vi "BKP-911x Power Supply_Create.vi"(0 "reference in":refnum<class "BKP-911x Power Supply.lvclass">, 2 "VISA resource name":refnum<visa-resource-name>, 3 "Serial Configuration":cluster{"Baud Rate":u32}={"Baud Rate"=9600} {"Baud Rate" items=["4800"=4800, "9600"=9600, "19200"=19200, "38400"=38400, "57600"=57600, "115200"=115200]}, 5 "error in (no error)":errorcluster) -> (13 "ProcessViRef":refnum<vi>, 14 "reference out":refnum<class "BKP-911x Power Supply.lvclass">, 19 "error out":errorcluster)   [LabVIEW 2018, in "BKP-911x Power Supply.lvclass"]
uses:
  BKP-911x Power Supply.lvclass
  controls/IO Signal List.ctl
  <instrlib>/BK Precision 911X Series/BK Precision 911X Series.lvlib
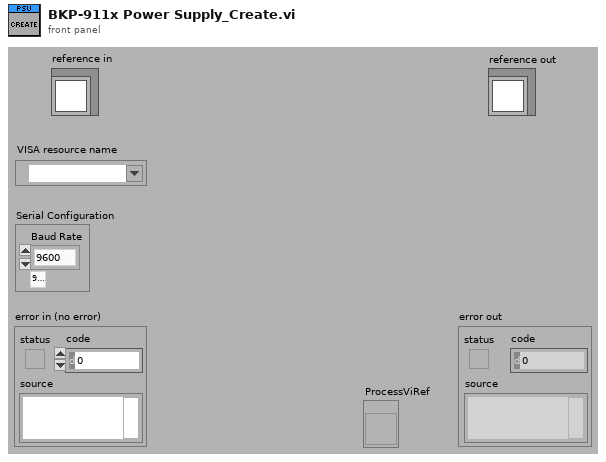
[diagram p1: front panel]
types:
  T1 = typedef "IO Signal List.ctl" = enum16{"Timestamp", "PSU_FB_U_VDC", "PSU_FB_I_AMP", "PSU_FB_W_WATT", "PSU_CMD_U_VDC", "PSU_CMD_I_AMP", "PSU_CMD_OUTPUT", "U_U_VDC", "V_U_VDC", "W_U_VDC", "U_I_AMP", "V_I_AMP", "W_I_AMP", "LCR_PRIMARY", "LCR_SECONDARY", "UV_R_mOhm", "UW_R_mOhm", "VW_R_mOhm", "UV_L_µH", "UW_L_µH", "VW_L_µH", "DIFF_UV_UW_L_µH", "DIFF_UV_VW_L_µH", "DIFF_UW_VW_L_µH", "DIFF_UV_UW_R_mOhm", "DIFF_UV_VW_R_mOhm", "DIFF_UW_VW_R_mOhm", "DIFF_UV_U_VDC", "DIFF_UW_U_VDC", "DIFF_VW_U_VDC", "PWM_CMD_DC_%", "PWM_CMD_VDC", "PWM_CMD_Hz", "PWM_FB_DC_%", "PWM_FB_VDC", "PWM_FB_Hz", "DO_RELAY_U_LCR_A", "DO_RELAY_V_LCR_A", "DO_RELAY_V_LCR_B", "DO_RELAY_W_LCR_B"}
  T2 = typedef "BKP-911x Power Supply.lvclass/ObjectAttributes.ctl" = cluster{"VISA resource name":refnum<visa-resource-name>, "Simulated?":bool, "Latest Values":dbl[], "Signal List":T1[], "Voltage Setpoint (V)":dbl, "Current Limit (A)":dbl, "Output Enabled?":bool}
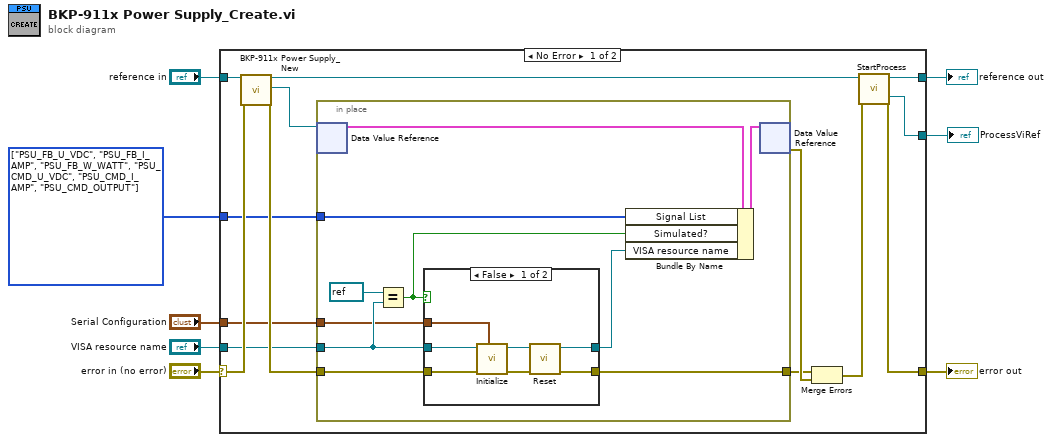
[diagram p0: block diagram]
diagram:
  w2 = T1[] [enum."PSU_FB_U_VDC", enum."PSU_FB_I_AMP", enum."PSU_FB_W_WATT", enum."PSU_CMD_U_VDC", enum."PSU_CMD_I_AMP", enum."PSU_CMD_OUTPUT"] items=["Timestamp", "PSU_FB_U_VDC", "PSU_FB_I_AMP", "PSU_FB_W_WATT", "PSU_CMD_U_VDC", "PSU_CMD_I_AMP", "PSU_CMD_OUTPUT", "U_U_VDC", "V_U_VDC", "W_U_VDC", "U_I_AMP", "V_I_AMP", "W_I_AMP", "LCR_PRIMARY", "LCR_SECONDARY", "UV_R_mOhm", "UW_R_mOhm", "VW_R_mOhm", "UV_L_µH", "UW_L_µH", "VW_L_µH", "DIFF_UV_UW_L_µH", "DIFF_UV_VW_L_µH", "DIFF_UW_VW_L_µH", "DIFF_UV_UW_R_mOhm", "DIFF_UV_VW_R_mOhm", "DIFF_UW_VW_R_mOhm", "DIFF_UV_U_VDC", "DIFF_UW_U_VDC", "DIFF_VW_U_VDC", "PWM_CMD_DC_%", "PWM_CMD_VDC", "PWM_CMD_Hz", "PWM_FB_DC_%", "PWM_FB_VDC", "PWM_FB_Hz", "DO_RELAY_U_LCR_A", "DO_RELAY_V_LCR_A", "DO_RELAY_V_LCR_B", "DO_RELAY_W_LCR_B"] ("Signal List")
  n1 = case shown="No Error" "error in (no error)" {
    selector: "error in (no error)" -> [w21 w43]
    tunnel: [w13 w43] -> w7
    tunnel: "reference in" -> [w22 w42]
    tunnel: [w15 w42] -> w5
    tunnel: "VISA resource name" -> [w12 _]
    tunnel: [w11 _] -> w3
    tunnel: w2 -> [w10 _]
    tunnel: "Serial Configuration" -> [w9 _]
    frame No Error {
      n2 = call "BKP-911x Power Supply_New.vi"("reference in"=w22, "error in (no error)"=w21) -> ("reference out"=w16:refnum<class "BKP-911x Power Supply.lvclass">, "DVRRefOut"=w19:refnum<data-value>, "error out"=w18:errorcluster)  [unwired: 14 in, 1 out]
      n3 = in-place {
        in-place-border: w18 -> [w30]
        in-place-border: [w29] -> w17
        in-place-border: w12 -> [w25]
        in-place-border: w10 -> [w28]
        in-place-border: w9 -> [w23]
        n4 = in-place-dvr #1(w19) -> (w31:T2)  [unwired: 1 out]
        n5 = Equal?(x=refnum<visa-resource-name> refnum ("VISA resource name"), y=w25) -> (x = y?=w24:bool)
        n6 = case shown="False" w24 {
          tunnel: w30 -> [w37 w40]
          tunnel: [w36 w40] -> w29
          tunnel: [w35 w41] -> w27
          tunnel: w25 -> [w34 w41]
          tunnel: w23 -> [w33 _]
          frame False {
            n7 = call <instrlib>:"Initialize.vi"("Serial Configuration"=w33, "error in (no error)"=w37, "VISA resource name"=w34) -> ("error out"=w38:errorcluster, "VISA resource name out"=w39:refnum<visa-resource-name>)  [unwired: 7 in]
            n8 = call <instrlib>:"Reset.vi"("error in (no error)"=w38, "VISA resource name"=w39) -> ("error out"=w36:errorcluster, "VISA resource name out"=w35:refnum<visa-resource-name>)  [unwired: 8 in]
          }
          frame True {
          }
        }
        n9 = Bundle By Name(cluster=w31, "Signal List"=w28, "Simulated?"=w24, "VISA resource name"=w27) -> (w32:T2)
        n10 = in-place-dvr #1(w32) -> (w20:errorcluster)  [unwired: 1 out]
      }
      n11 = Merge Errors(w17, w20) -> (w14:errorcluster)
      n12 = call "StartProcess.vi"("reference in"=w16, "error in (no error)"=w14) -> ("reference out"=w15:refnum<class "BKP-911x Power Supply.lvclass">, "ProcessViRef"=w11:refnum<vi>, "error out"=w13:errorcluster)  [unwired: 13 in, 2 out]
    }
    frame Error {
      # "VI-TechBaseTemplate_Simple_6x8x6"
    }
  }
  "error out" <- w7
  "reference out" <- w5
  "ProcessViRef" <- w3
